vi "WSVCAP SHL Host LL Set Read_Write Parameters.vi"(0 "Transaction":T2, 1 "Wait Ticks":u32, 2 "Slave Address":u8, 5 "Bytes":u8, 7 "Sub Address [U8]":u8=191 format="%.0x", 9 "Socket Mask [U64]":u64=1 format="%016x", 11 "error in (no error)":errorcluster, 12 "UUT Set (0/1)":u8, 14 "FPGA":T1) -> (15 "error out":errorcluster)   [LabVIEW 2017]
uses:
  Type Defs/WSVCAP SHL Transaction Enum.ctl
  Type Defs/WSVCAP SHL FPGA Enum.ctl
  Type Defs/WSVCAP SHL Top Level Control Operation Enum.ctl
  Type Defs/WSVCAP SHL State.ctl
  Type Defs/WSVCAP SHL Top Level Control Enum.ctl
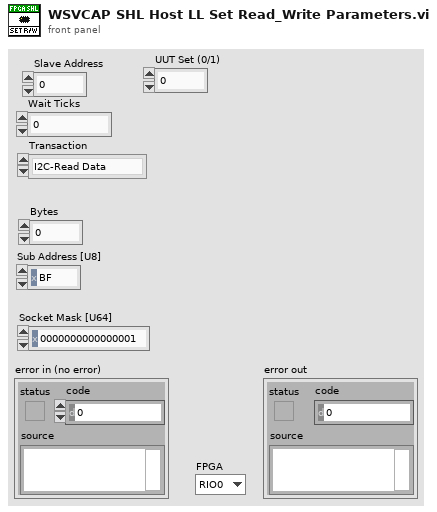
[diagram p1: front panel]
types:
  T1 = typedef "WSVCAP SHL FPGA Enum.ctl" = enum16{"RIO0", "RIO1"}
  T2 = typedef "WSVCAP SHL Transaction Enum.ctl" = enum16{"I2C-Read Data", "I2C-Write Data", "RFFE-Ext Write", "RFFE-Ext Read"}
  T3 = typedef "WSVCAP SHL Top Level Control Enum.ctl" = enum16{"Start", "Cmd", "Transaction", "Wait Ticks", "Socket Mask", "UUT Set", "Slave Address", "Sub Address", "Bytes to Write", "Bytes to Read", "Write Data", "Write Flag", "Read Data", "Read Flag", "Ack Read", "Read Status Flag", "Ack Read Status", "Status", "Cycle Count", "Stop Cycle", "Exit"}
  T4 = typedef "WSVCAP SHL State.ctl" = enum8{"Idle", "Transfer Data"}
  T5 = typedef "WSVCAP SHL Top Level Control Operation Enum.ctl" = enum16{"Initialize", "Set Control", "Read Control", "Close"}
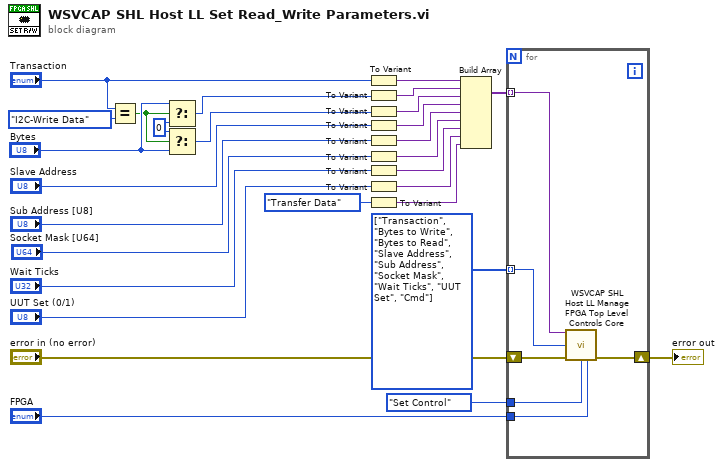
[diagram p0: block diagram]
diagram:
  w19 = u8 0 ("t")
  w21 = T3[] [enum."Transaction", enum."Bytes to Write", enum."Bytes to Read", enum."Slave Address", enum."Sub Address", enum."Socket Mask", enum."Wait Ticks", enum."UUT Set", enum."Cmd"] items=["Start", "Cmd", "Transaction", "Wait Ticks", "Socket Mask", "UUT Set", "Slave Address", "Sub Address", "Bytes to Write", "Bytes to Read", "Write Data", "Write Flag", "Read Data", "Read Flag", "Ack Read", "Read Status Flag", "Ack Read Status", "Status", "Cycle Count", "Stop Cycle", "Exit"]
  n1 = Equal?(x="Transaction", y=WSVCAP_SHL_Transaction_Enum."I2C-Write Data" ("Transaction")) -> (x = y?=w13:bool)
  n2 = Select(t="Bytes", s=w13, f=w19) -> (s? t:f=w18:u8)
  n3 = Select(t=w19, s=w13, f="Bytes") -> (s? t:f=w17:u8)
  n4 = To Variant(anything="Transaction") -> (Variant=w27:variant)
  n5 = To Variant(anything=w18) -> (Variant=w26:variant)
  n6 = To Variant(anything=w17) -> (Variant=w16:variant)
  n7 = To Variant(anything="Slave Address") -> (Variant=w4:variant)
  n8 = To Variant(anything="Sub Address [U8]") -> (Variant=w12:variant)
  n9 = To Variant(anything="Socket Mask [U64]") -> (Variant=w11:variant)
  n10 = To Variant(anything="Wait Ticks") -> (Variant=w7:variant)
  n11 = To Variant(anything="UUT Set (0/1)") -> (Variant=w2:variant)
  n12 = To Variant(anything=WSVCAP_SHL_State."Transfer Data" ("SPI_Cmd")) -> (Variant=w22:variant)
  n13 = Build Array(w27, w26, w16, w4, w12, w11, w7, w2, w22) -> (w25:variant[])
  n14 = for {
    tunnel: WSVCAP_SHL_Top_Level_Control_Operation_Enum."Set Control" ("Operation") -> [w34]
    tunnel: w25 -> [w33] mode=indexing
    tunnel: w21 -> [w32] mode=indexing
    shift-right: [w30] -> w23
    shift-left: "error in (no error)" -> [w31]
    tunnel: "FPGA" -> [w29]
    n15 = call "WSVCAP SHL Host LL Manage FPGA Top Level Controls Core.vi"("Value In"=w33, "FPGA Top Level Control"=w32, "error in (no error)"=w31, "Operation"=w34, "FPGA"=w29) -> ("error out"=w30:errorcluster)  [unwired: 9 in, 1 out]
  }
  "error out" <- w23
